vi "CIMAQ_Sub_BoundingCircle.vi"(7 "error in (no error)":errorcluster, 10 "In":T1) -> (0 "error out":errorcluster, 1 "Radius":dbl, 2 "Center":cluster{i32, i32}, 3 "Out":T1)   [LabVIEW 2017]
uses:
  <vilib>/vision/Image Controls.llb/IMAQ Image.ctl
  <vilib>/vision/NI_Vision_Development_Module.lvlib
  <vilib>/Analysis/NI_AAL_Geometry.lvlib
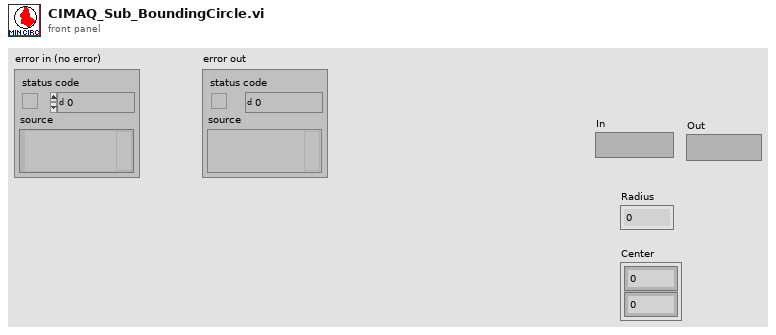
[diagram p1: front panel]
types:
  T1 = typedef "IMAQ Image.ctl" = refnum<image>
  T2 = enum32{"AutoM", "Close", "Dilate", "Erode", "Gradient", "Gradient out", "Gradient in", "Hit miss", "Open", "PClose", "POpen", "Thick", "Thin"}
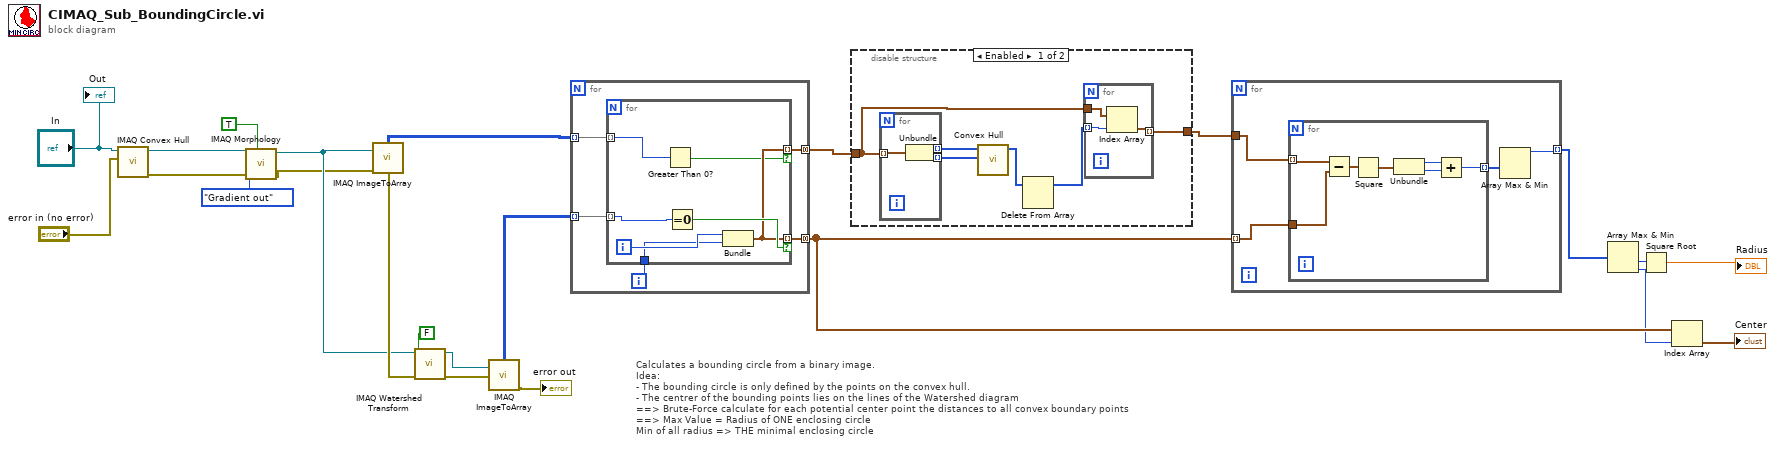
[diagram p0: block diagram]
diagram:
  # "Calculates a bounding circle from a binary image.\nIdea:\n- The bounding circle is only defined by the points on the convex hull. \n- The centrer of the bounding points lies on the lines of the Watershed diagram\n==> Brute-Force calculate for each potential center point the distances to all convex boundary points \n==> Max Value = Radius of ONE enclosing circle\nMin of all radius => THE minimal enclosing circle"
  n1 = call "IMAQ Convex Hull"("error in (no error)"="error in (no error)", "Image Src"="In") -> ("error out"=w5:errorcluster, "Image Dst Out"=w7:T1)  [unwired: 8 in]
  n2 = call "IMAQ Morphology"("Square/Hexa (Square)"=TRUE, "error in (no error)"=w5, "Operation"=T2."Gradient out", "Image Src"=w7) -> ("error out"=w4:errorcluster, "Image Dst Out"=w12:T1)  [unwired: 6 in]
  n3 = call "IMAQ ImageToArray"("error in (no error)"=w4, "Image"=w12) -> ("error out"=w13:errorcluster, "Image Pixels (U8)"=w11:u8[][])  [unwired: 2 in, 3 out]
  n4 = call "IMAQ Watershed Transform"("error in (no error)"=w13, "Connectivity 4/8 (8)"=FALSE, "Image Src"=w12) -> ("error out"=w3:errorcluster, "Image Dst Out"=w18:T1)  [unwired: 6 in, 1 out]
  n5 = call "IMAQ ImageToArray"("error in (no error)"=w3, "Image"=w18) -> ("error out"=→"error out":errorcluster, "Image Pixels (U8)"=w10:u8[][])  [unwired: 2 in, 3 out]
  n6 = for {
    tunnel: w10 -> [w28] mode=indexing
    tunnel: [w26] -> w22 mode=concatenating
    tunnel: w11 -> [w25] mode=indexing
    tunnel: [w24] -> w16 mode=concatenating
    i -> [w27]
    n7 = for {
      tunnel: w28 -> [w29] mode=indexing
      tunnel: w27 -> [w34]
      tunnel: [w31] -> w26 mode=indexing if=w33
      tunnel: w25 -> [w32] mode=indexing
      tunnel: [w31] -> w24 mode=indexing if=w30
      i -> [w35]
      n8 = Greater Than 0?(x=w32) -> (x > 0?=w30:bool)
      n9 = Equal To 0?(x=w29) -> (x = 0?=w33:bool)
      n10 = Bundle(w35, w34) -> (w31:cluster{i32, i32})  [unwired: 1 in]
    }
  }
  n11 = disable-structure shown="Enabled" {
    disable-tunnel: w16 -> [w39 w48]
    disable-tunnel: [w38 w48] -> w17
    frame Enabled {
      n12 = for {
        tunnel: w39 -> [w47] mode=indexing
        tunnel: [w46] -> w41 mode=indexing
        tunnel: [w45] -> w40 mode=indexing
        n13 = Unbundle(w47) -> (w46:i32, w45:i32)
      }
      n14 = call <vilib>:"Convex Hull.vi"("Y"=w40, "X"=w41) -> ("Convex Hull"=w37:i32[])  [unwired: 8 in, 1 out]
      n15 = Delete From Array(array=w37) -> (array with subset deleted=w36:i32[])  [unwired: 2 in, 1 out]
      n16 = for {
        tunnel: w36 -> [w44] mode=indexing
        tunnel: w39 -> [w43]
        tunnel: [w42] -> w38 mode=indexing
        n17 = Index Array(array=w43, index=w44) -> (element=w42:cluster{i32, i32})
      }
    }
    frame Disabled {
      # "The LabVIEW Convex Hull Algorithm reduces the\npixels even more. Reduces computational load!"
    }
  }
  n18 = for {
    tunnel: [w50] -> w19 mode=indexing
    tunnel: w22 -> [w52] mode=indexing
    tunnel: w17 -> [w51]
    n19 = for {
      tunnel: w52 -> [w54]
      tunnel: w51 -> [w55] mode=indexing
      tunnel: [w53] -> w49 mode=indexing
      n20 = Subtract(x=w55, y=w54) -> (x-y=w59:cluster{i32, i32})
      n21 = Square(x=w59) -> (x^2=w58:cluster{i32, i32})
      n22 = Unbundle(w58) -> (w57:i32, w56:i32)
      n23 = Add(x=w57, y=w56) -> (x+y=w53:i32)
    }
    n24 = Array Max & Min(array=w49) -> (max value=w50:i32)  [unwired: 3 out]
  }
  n25 = Array Max & Min(array=w19) -> (min value=w14:i32, min index (indices)=w15:i32)  [unwired: 2 out]
  n26 = Square Root(x=w14) -> (sqrt(x)=→"Radius":dbl)
  n27 = Index Array "Index Array"(array=w22, index=w15) -> (element=→"Center":cluster{i32, i32})
  "Out" <- "In"
